vi "MH_Graph_Binned.vi"() -> ()   [LabVIEW 2019]
panel:
  in  "Average size":i32=1
  out "Numérique":i32
  out "Correlations Out":dbl[][](array[numeric])
  out "Graph":dbl[][](graph)
  in  "BinSize":u32=1
  in  "Correlations":u32[](array[numeric])
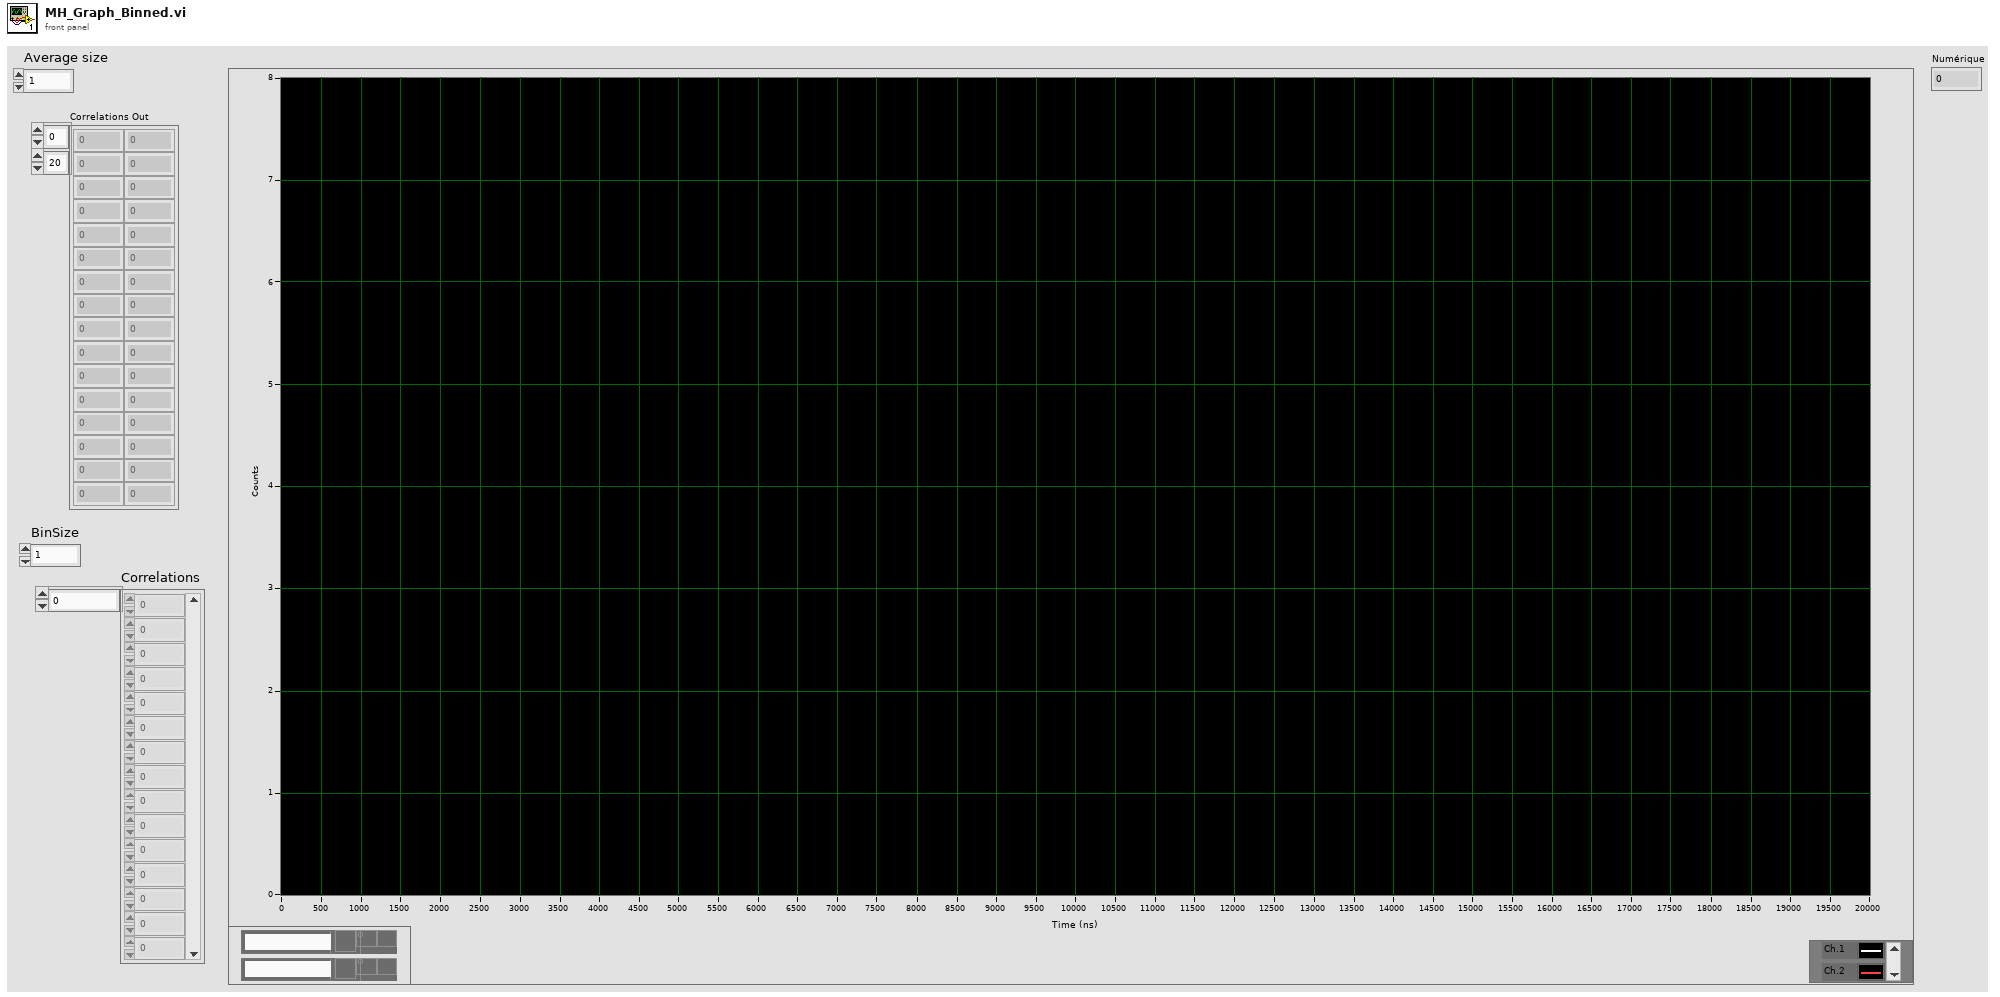
[diagram p1: front panel]
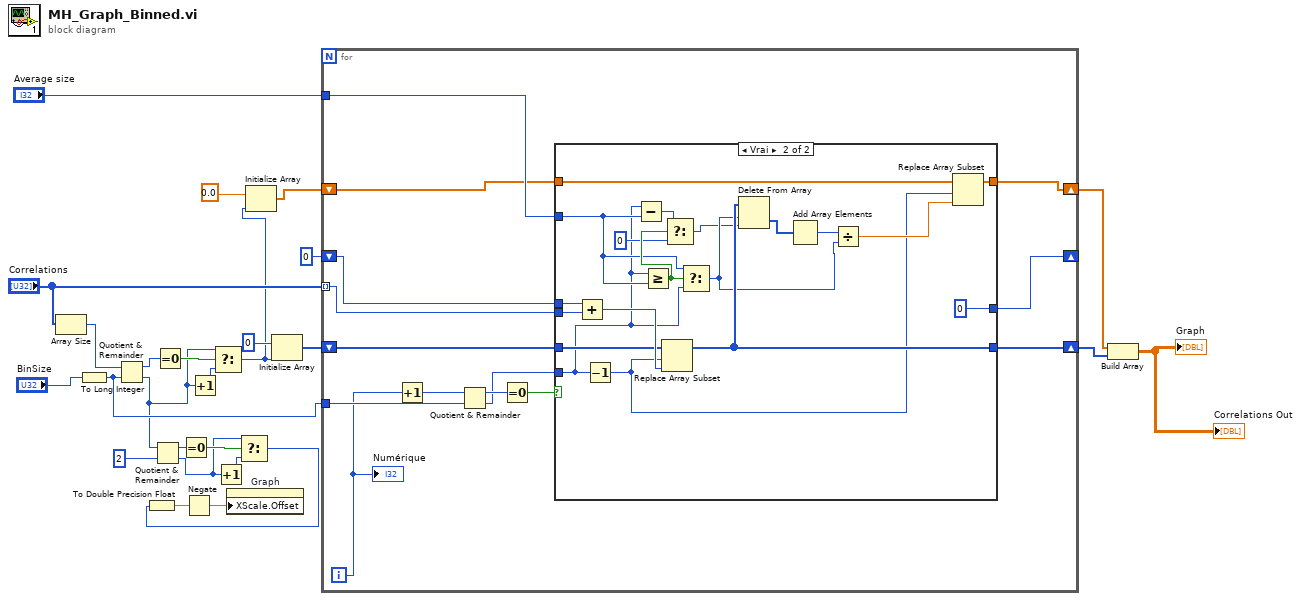
[diagram p0: block diagram]
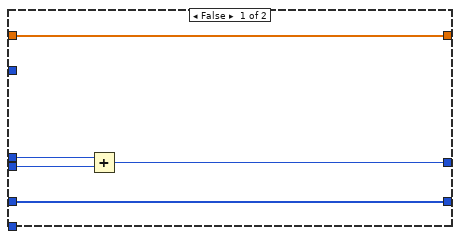
[diagram p2: hidden frame]
diagram:
  n1 = Array Size(array="Correlations") -> (size(s)=w16:i32)
  n2 = To Long Integer(number="BinSize") -> (32bit integer=w19:i32)
  n3 = Quotient & Remainder(x=w16, y=w19) -> (x-y*floor(x/y)=w22:i32, floor(x/y)=w15:i32)
  n4 = Quotient & Remainder(x=w15, y=2) -> (x-y*floor(x/y)=w11:i32, floor(x/y)=w10:i32)
  n5 = Equal To 0?(x=w22) -> (x = 0?=w21:bool)
  n6 = Equal To 0?(x=w11) -> (x = 0?=w13:bool)
  n7 = Increment(x=w15) -> (x+1=w20:i32)
  n8 = Select(t=w15, s=w21, f=w20) -> (s? t:f=w4:i32)
  n9 = Increment(x=w10) -> (x+1=w12:i32)
  n10 = Select(t=w10, s=w13, f=w12) -> (s? t:f=w9:i32)
  n11 = To Double Precision Float(number=w9) -> (double precision float=w18:dbl)
  n12 = Negate(x=w18) -> (-x=w17:dbl)
  n13 = property on="Graph" class="GraphWF (strict)"("XScale.Offset"=w17) -> ()  [unwired: 2 in, 2 out]
  n14 = Initialize Array(0.0 ("x/y"), w4) -> (w3:dbl[])
  n15 = Initialize Array(u32 0 ("Correlations"), w4) -> (w7:u32[])
  n16 = for {
    tunnel: "Correlations" -> [w37] mode=indexing
    tunnel: w19 -> [w40]
    shift-right: [w36] -> _
    shift-left: u32 0 -> [w35]
    shift-right: [w33] -> w1
    shift-left: w7 -> [w31]
    tunnel: "Average size" -> [w30]
    shift-right: [w27] -> w2
    shift-left: w3 -> [w28]
    i -> [w29]
    n17 = Increment(x=w29) -> (x+1=w32:i32)
    n18 = Quotient & Remainder(x=w32, y=w40) -> (x-y*floor(x/y)=w39:i32, floor(x/y)=w34:i32)
    n19 = Equal To 0?(x=w39) -> (x = 0?=w38:bool)
    n20 = case shown="Vrai" w38 {
      tunnel: w37 -> [w45 w62]
      tunnel: [w44 u32 0] -> w36
      tunnel: w35 -> [w43 w63]
      tunnel: w31 -> [w42 w58]
      tunnel: w34 -> [_ w48]
      tunnel: [w42 w57] -> w33
      tunnel: w30 -> [_ w50]
      tunnel: w28 -> [w41 w56]
      tunnel: [w41 w55] -> w27
      frame False {
        n21 = Add(x=w43, y=w45) -> (x+y=w44:u32)
      }
      frame True {
        n22 = Add(x=w63, y=w62) -> (x+y=w61:u32)
        n23 = Decrement(x=w48) -> (x-1=w47:i32)
        n24 = Subtract(x=w48, y=w50) -> (x-y=w49:i32)
        n25 = Greater Or Equal?(x=w48, y=w50) -> (x >= y?=w52:bool)
        n26 = Replace Array Subset(array=w58, new element=w61, index=w47) -> (w57:u32[])
        n27 = Select(t=w49, s=w52, f=0 ("cas faux")) -> (s? t:f=w46:i32)
        n28 = Select(t=w50, s=w52, f=w48) -> (s? t:f=w53:i32)
        n29 = Delete From Array(array=w57, length=w53, index=w46) -> (deleted portion=w60:u32[])  [unwired: 1 out]
        n30 = Add Array Elements(numeric array=w60) -> (sum=w59:u32)
        n31 = Divide(x=w59, y=w53) -> (x/y=w54:dbl)
        n32 = Replace Array Subset(array=w56, new element=w54, index=w47) -> (w55:dbl[])
      }
    }
    "Numérique" <- w29
  }
  n33 = Build Array(w2, w1) -> (→"Graph" →"Correlations Out":dbl[][])
